vi "Set Position via Global Variables.vi"(1 "Position":dbl) -> ()   [LabVIEW 2013]
uses:
  PPMS Global.vi
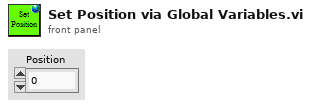
[diagram p1: front panel]
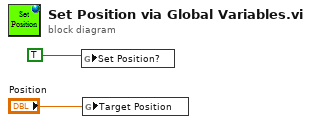
[diagram p0: block diagram]
diagram:
  n1 = global write "PPMS Global.vi" "Set Position?"(TRUE ("Set Position?")) -> ()
  n2 = global write "PPMS Global.vi" "Target Position"("Position") -> ()
